vi "Prepare Control.vi"(7 "VolatusAPI":refnum<class "VolatusAPI.lvclass">, 8 "error in (no error)":errorcluster, 11 "SequencedValves in":refnum<class "TriggerDelayControl.lvclass">) -> (0 "error out":errorcluster, 3 "SequencedValves out":refnum<class "TriggerDelayControl.lvclass">)   [LabVIEW 2020, in "VolatusControl.lvlib" / "TriggerDelayControl.lvclass"]
uses:
  TriggerDelayControl.lvclass
  Volatus/VolatusAPI/VolatusAPI.lvclass
  TriggerDelayControl.lvclass/TriggerDelayControl.ctl
  Volatus/Module Identity/Module Identity.lvclass/Module Identity.ctl
  Volatus/Module Identity/Create.vi
  Volatus/Module Identity/Module Identity.lvclass
  C:/dev/lv20CE/relink/lv-volatus/Volatus/Identity/Identity.lvclass
  Volatus/VolatusAPI/Lookup Q.vi
  lv-vecto/Vecto/Group/Group.lvclass
  lv-vecto/Vecto/StringGroup/StringGroup.lvclass
  lv-vecto/Vecto/GroupAbstract/GroupAbstract.lvclass
  C:/dev/lv20CE/relink/lv-vecto/Vecto/GroupAbstract/GroupAbstract.lvclass
  C:/dev/lv20CE/relink/lv-vecto/Vecto/StringGroup/StringGroup.lvclass
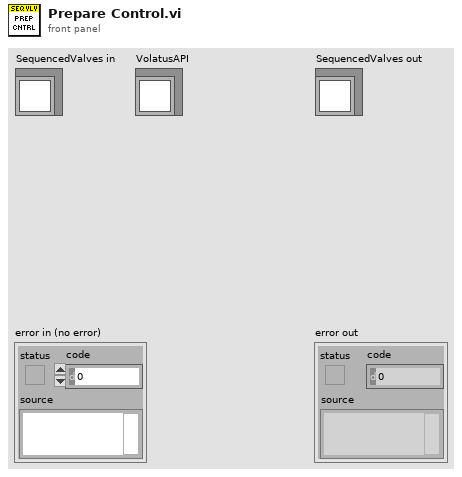
[diagram p1: front panel]
types:
  T1 = typedef "VolatusControl.lvlib/TriggerDelayControl.lvclass/Channel Type.ctl" = enum16{"Double", "String"}
  T2 = typedef "VectoConfig.lvlib/Channel Info.ctl" = cluster{"Name":string, "Group":string, "Owning Node":string, "Owning Task":string, "Resource":string}
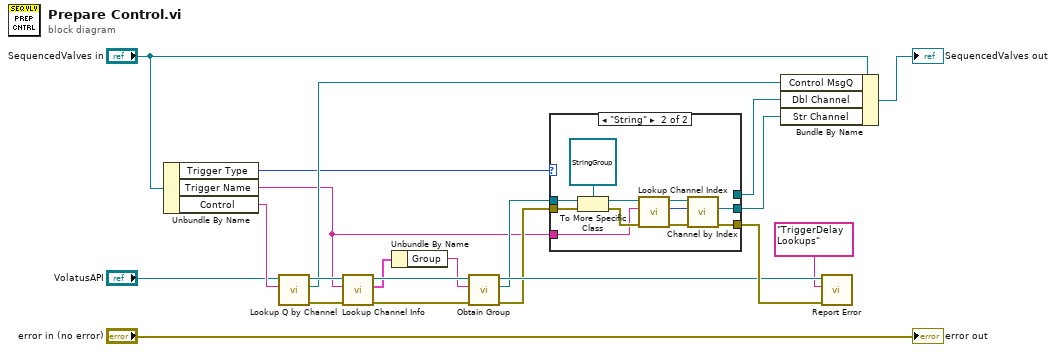
[diagram p0: block diagram]
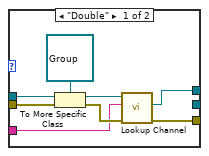
[diagram p2: hidden frame]
diagram:
  n1 = Unbundle By Name("SequencedValves in") -> ("Trigger Type"=w6:T1, "Trigger Name"=w3:string, "Control"=w18:string)
  n2 = call "Lookup Q by Channel.vi"("Channel Name"=w18, "VolatusAPI in"="VolatusAPI") -> ("error out"=w16:errorcluster, "MessageQ"=w13:refnum<class "MessageQ.lvclass">, "VolatusAPI out"=w17:refnum<class "VolatusAPI.lvclass">)  [unwired: 7 in]
  n3 = call "Lookup Channel Info.vi"("error in (no error)"=w16, "Channel Name"=w3, "VolatusAPI in"=w17) -> ("error out"=w10:errorcluster, "Channel Info"=w9:T2, "VolatusAPI out"=w12:refnum<class "VolatusAPI.lvclass">)  [unwired: 5 in, 1 out]
  n4 = Unbundle By Name(w9) -> ("Group"=w11:string)
  n5 = call "Obtain Group.vi"("error in (no error)"=w10, "Group Name"=w11, "VolatusAPI in"=w12) -> ("error out"=w4:errorcluster, "Group"=w5:refnum<class "GroupAbstract.lvclass">, "VolatusAPI out"=w8:refnum<class "VolatusAPI.lvclass">)  [unwired: 6 in]
  n6 = case shown="\"String\"" w6 {
    tunnel: w5 -> [w29 w40]
    tunnel: w4 -> [w27 w38]
    tunnel: w3 -> [w24 w35]
    tunnel: [w23 _] -> w2
    tunnel: [w22 w31] -> w21
    tunnel: [_ w30] -> w1
    frame "Double" {
      n7 = To More Specific Class(target class=refnum<class "Group.lvclass"> refnum ("Vecto.lvlib:Group.lvclass"), reference=w29, error in=w27) -> (specific class reference=w26:refnum<class "Group.lvclass">, error out=w25:errorcluster)
      n8 = call "Lookup Channel.vi"("error in (no error)"=w25, "Channel Name"=w24, "Group in"=w26) -> ("error out"=w22:errorcluster, "Channel"=w23:refnum<class "Channel.lvclass">)  [unwired: 6 in, 1 out]
    }
    frame "String" {
      n9 = To More Specific Class(target class=refnum<class "StringGroup.lvclass"> refnum ("Vecto.lvlib:StringGroup.lvclass"), reference=w40, error in=w38) -> (specific class reference=w37:refnum<class "StringGroup.lvclass">, error out=w36:errorcluster)
      n10 = call "Lookup Channel Index.vi"("error in (no error)"=w36, "Channel Name"=w35, "GroupAbstract in"=w37) -> ("error out"=w33:errorcluster, "Index"=w32:i32, "GroupAbstract out"=w34:refnum<class "StringGroup.lvclass">)  [unwired: 6 in]
      n11 = call "Channel by Index.vi"("error in (no error)"=w33, "Index"=w32, "StringGroup in"=w34) -> ("error out"=w31:errorcluster, "StringChannel"=w30:refnum<class "StringChannel.lvclass">)  [unwired: 6 in, 1 out]
    }
  }
  n12 = Bundle By Name(cluster="SequencedValves in", "Control MsgQ"=w13, "Dbl Channel"=w2, "Str Channel"=w1) -> (→"SequencedValves out":refnum<class "TriggerDelayControl.lvclass">)
  n13 = call "Report Error.vi"("error in (no error)"=w21, "Context"="TriggerDelay Lookups", "VolatusAPI in"=w8) -> ()  [unwired: 7 in, 2 out]
  "error out" <- "error in (no error)"
